vi "TCP Tester.vi"() -> ()   [LabVIEW 2019]
uses:
  <userlib>/Jet Engineering/JET_QSM/Code/Private/JET_QSM - Add State [String API].vi
  <userlib>/Jet Engineering/JET_QSM/Code/Private/JET_QSM_InvalidOption STYP.ctl
  Code/Shared/Map/Map.lvclass
panel:
  out "Recent states before Error (with tick counts) 3":string="0.167 sec ago: VI Initialize\n0.167 sec ago: Window Open\n0.110 sec ago: Control Update\n0.110 sec ago: Indicator Update\n0.000 sec ago: Error Handler\r\n"
  in  "Status 2":T1
  out "error out 2":errorcluster
  in  "Port":u16
  in  "IP Address":string
  out "Recent states before Error (with tick counts) 2":string="0.167 sec ago: VI Initialize\n0.167 sec ago: Window Open\n0.110 sec ago: Control Update\n0.110 sec ago: Indicator Update\n0.000 sec ago: Error Handler\r\n"
  in  "Status":T2
  out "error out":errorcluster
  in  "stop":bool
  in  "Send Button":bool
  out "Received Message":string
  in  "Message to Send":string
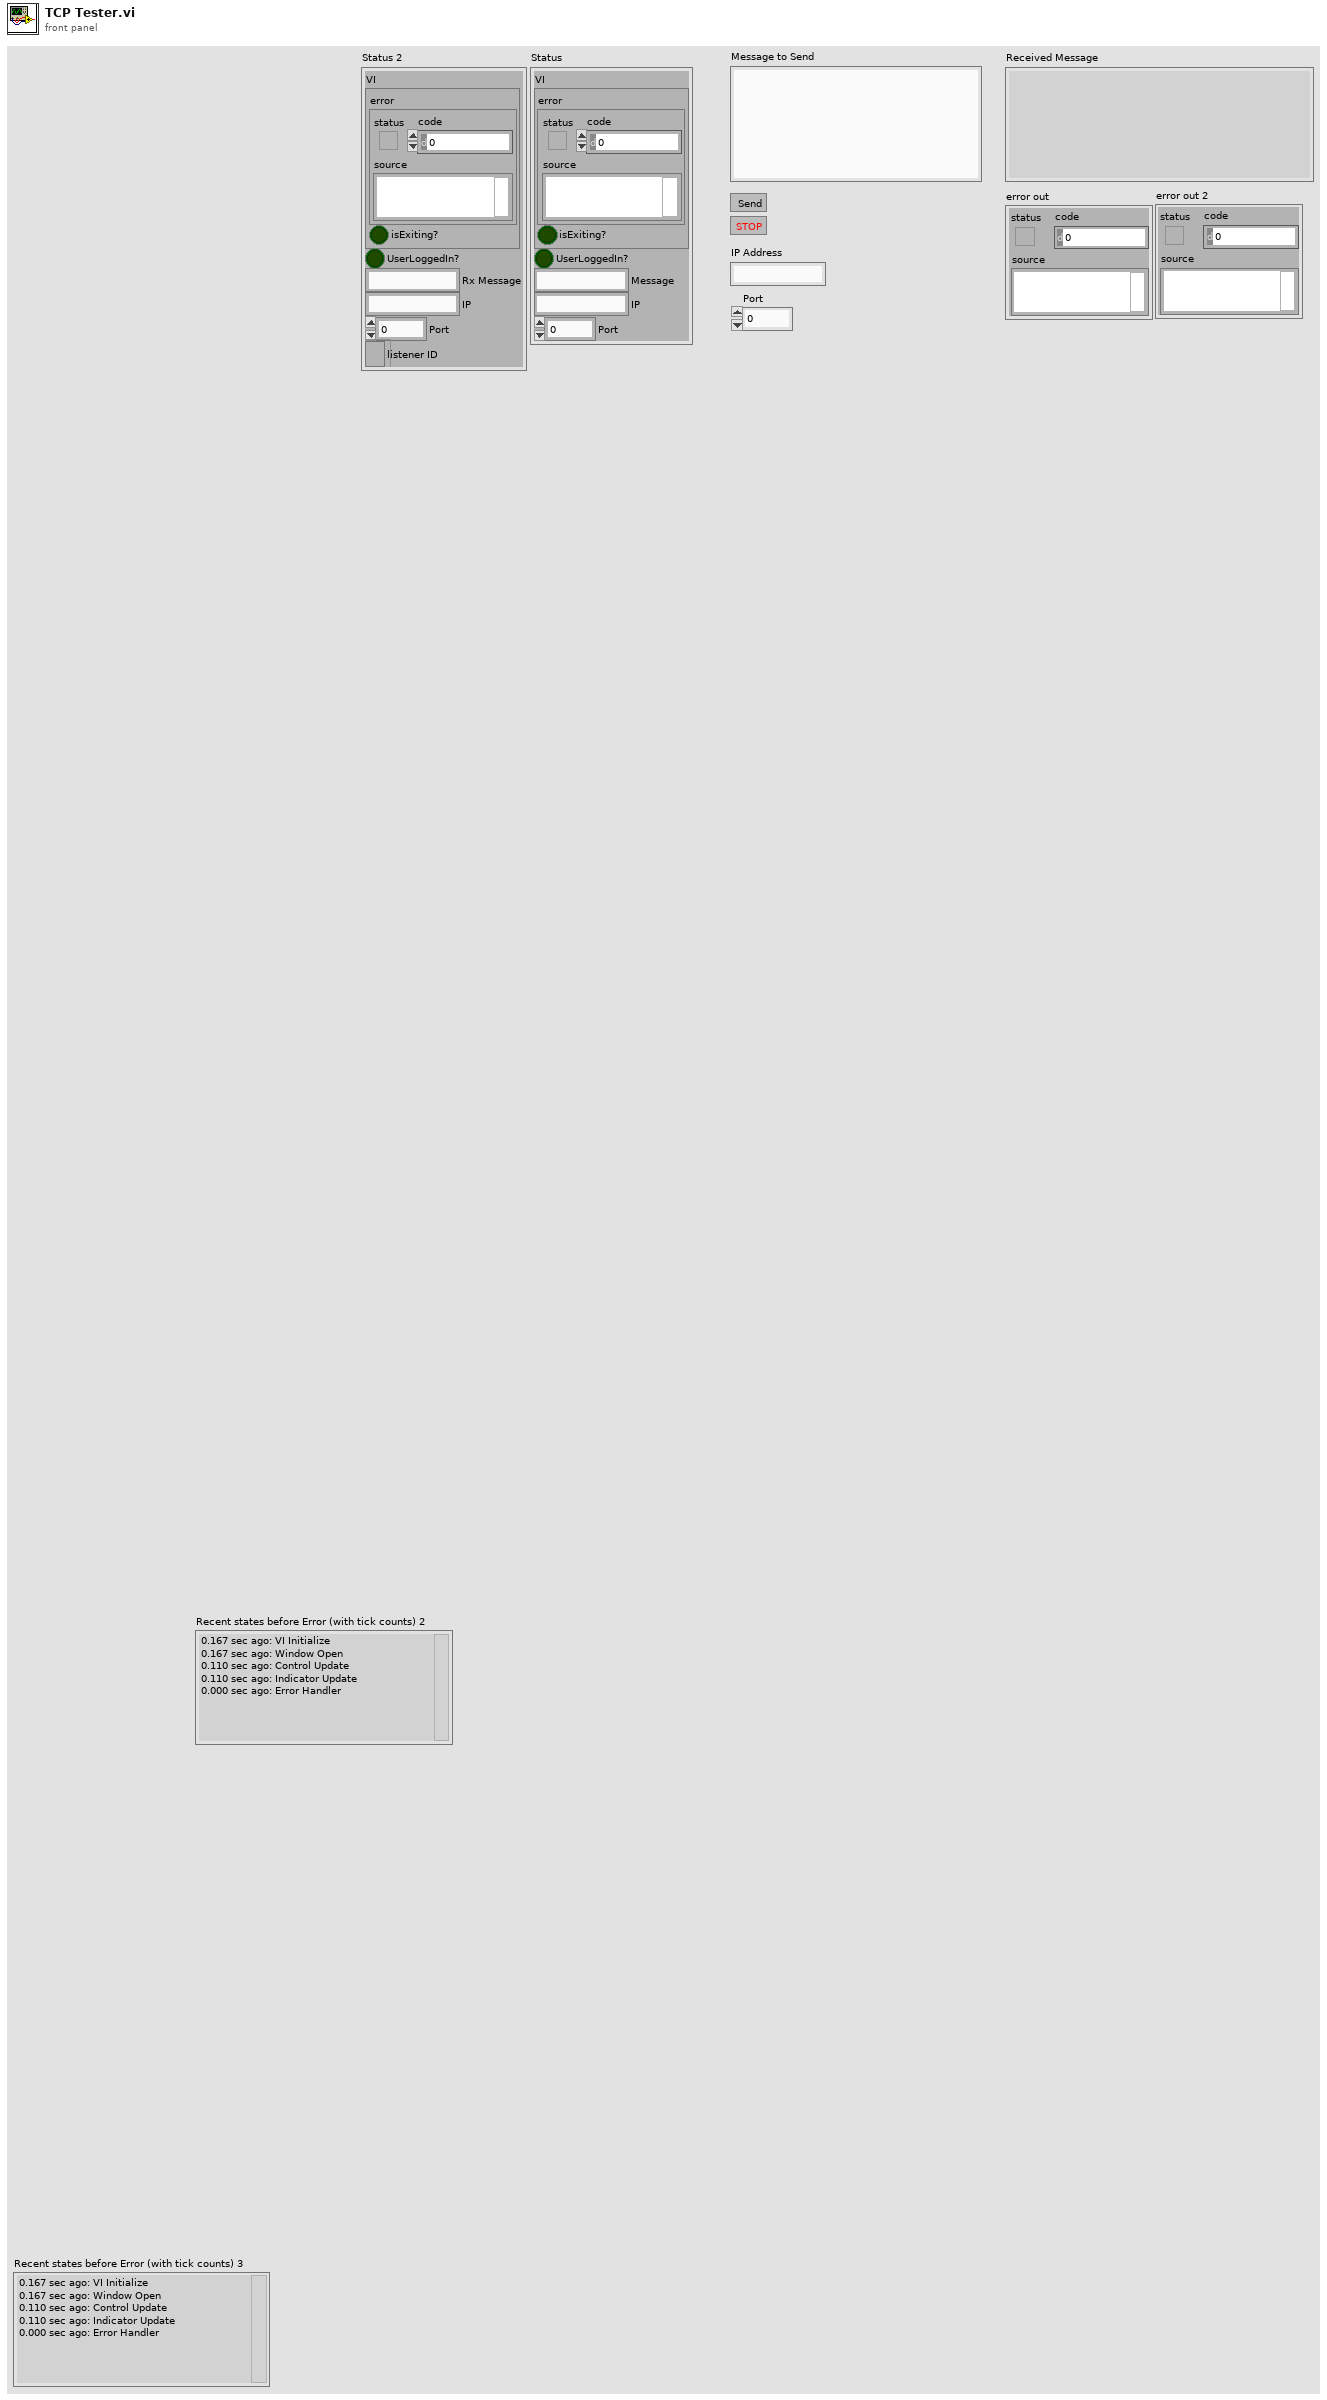
[diagram p1: front panel]
types:
  T1 = cluster{"VI":cluster{"error":errorcluster, "isExiting?":bool}, "UserLoggedIn?":bool, "Rx Message":string, "IP":string, "Port":u16, "listener ID":refnum<k5>}
  T2 = cluster{"VI":cluster{"error":errorcluster, "isExiting?":bool}, "UserLoggedIn?":bool, "Message":string, "IP":string, "Port":u16}
  T3 = typedef "JET_QSM_InvalidOption STYP.ctl" = enum16{"Ignore", "Dialog", "Error"}
  T4 = typedef "JET_QSM_Refnum STYP.ctl" = cluster{"state":cluster{"queue":refnum<queue>, "idle":string, "error":string, "STOP":string}, "debug":cluster{"enabled?":bool, "queue":refnum<queue>}, "Invalid.option":T3, "QSM.Name":string}
  T5 = enum32{"invalid app kind", "Development System", "Run Time System", "Student Edition", "Embedded LabVIEW", "Evaluation", "Custom"}
  T6 = typedef "JET_QSM_Element STYP.ctl" = cluster{"state":string, "data":variant, "comment":string}
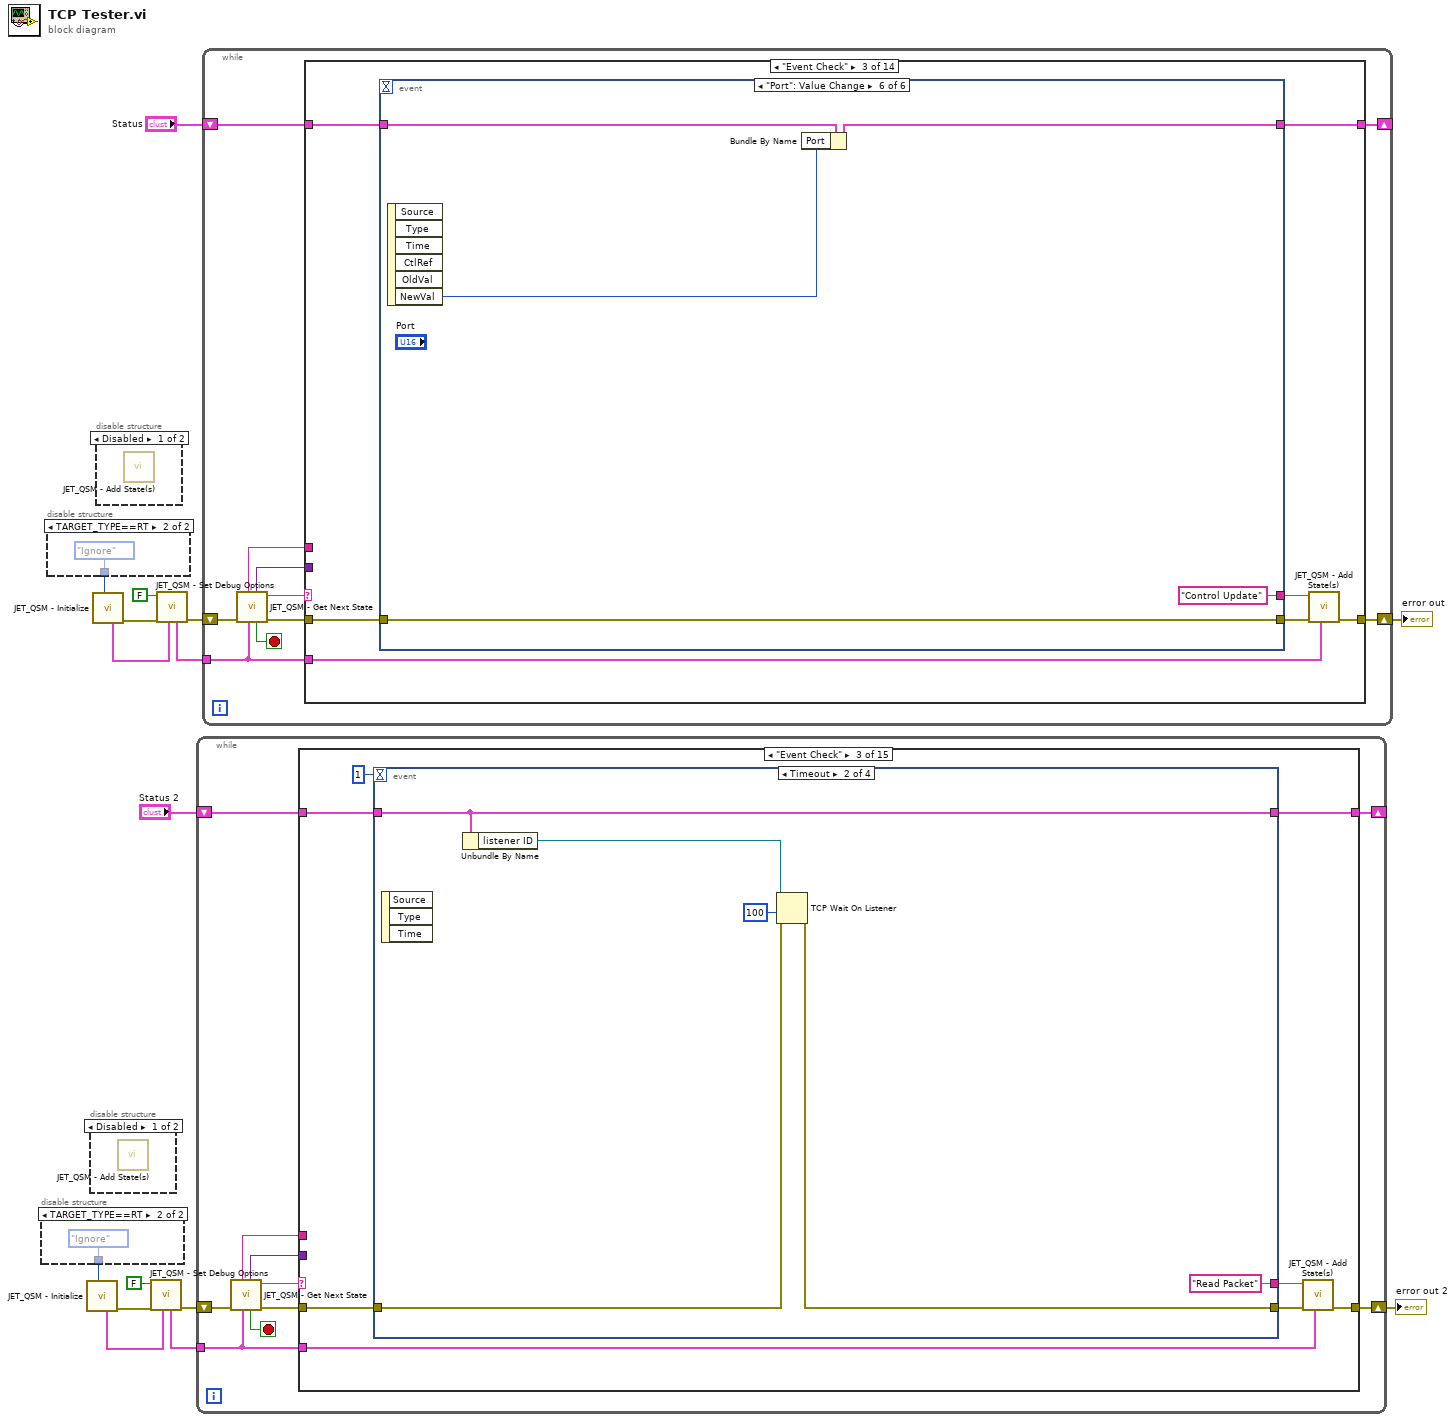
[diagram p0: block diagram]
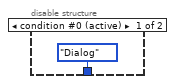
[diagram p2: hidden frame]
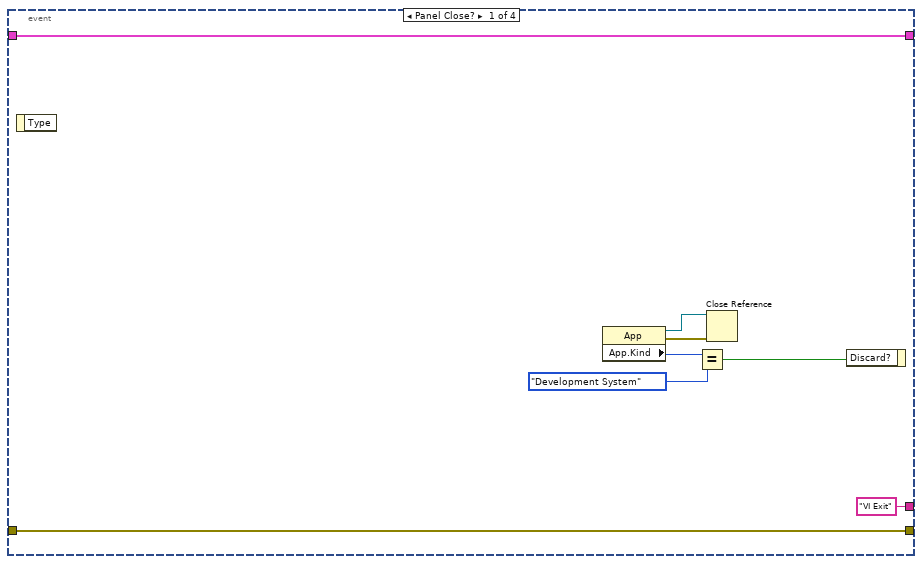
[diagram p6: hidden frame]
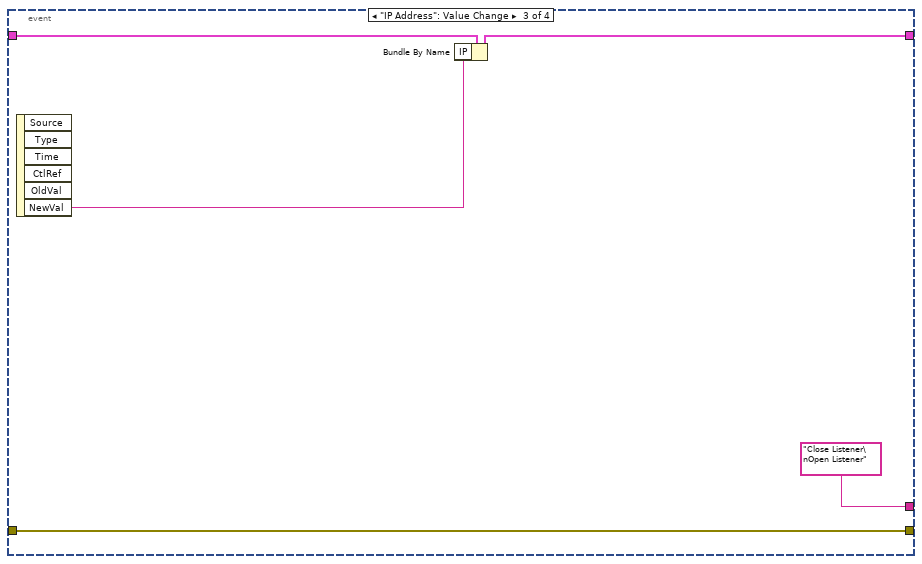
[diagram p7: hidden frame]
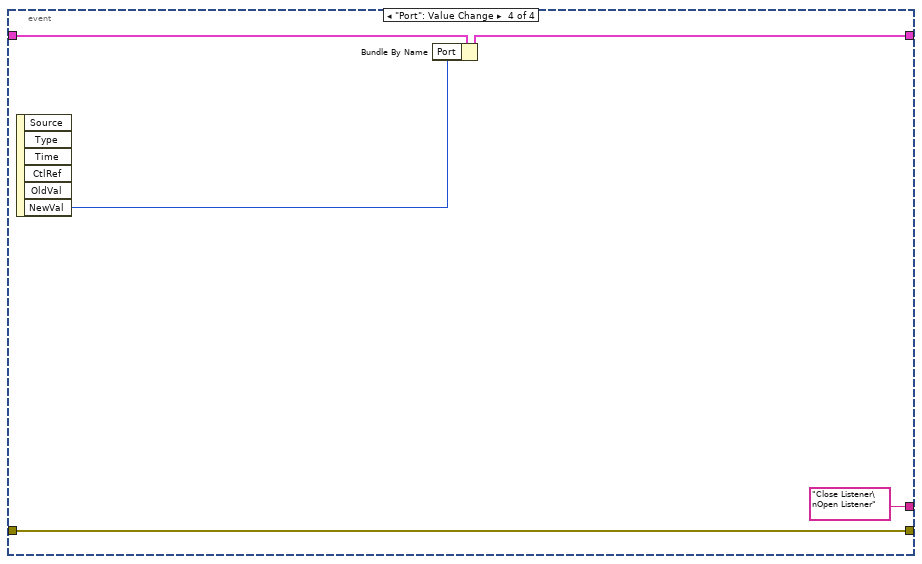
[diagram p8: hidden frame]
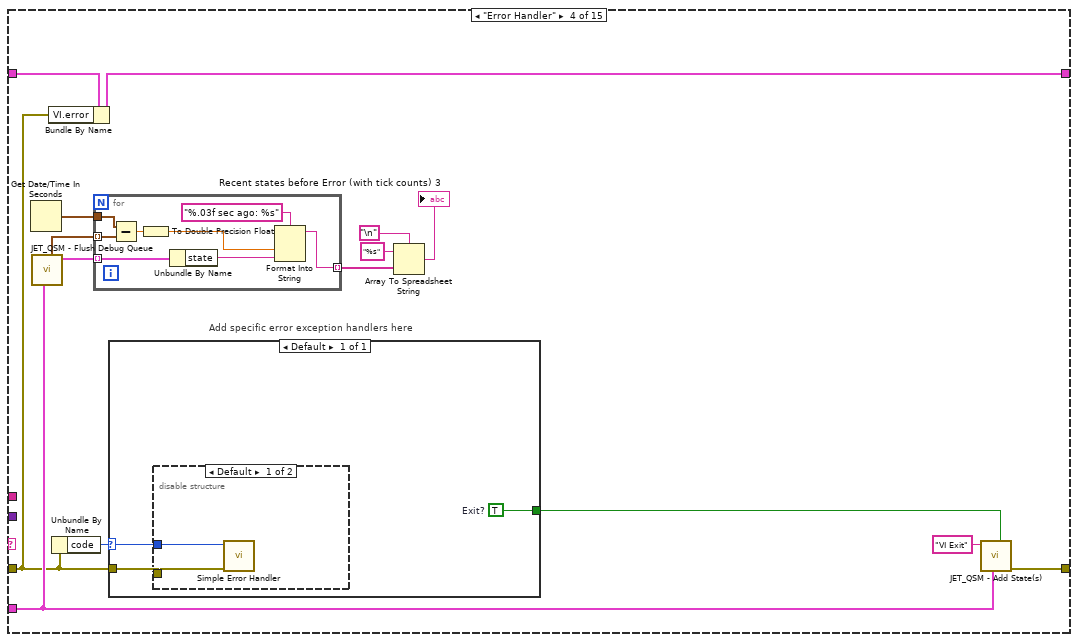
[diagram p9: hidden frame]
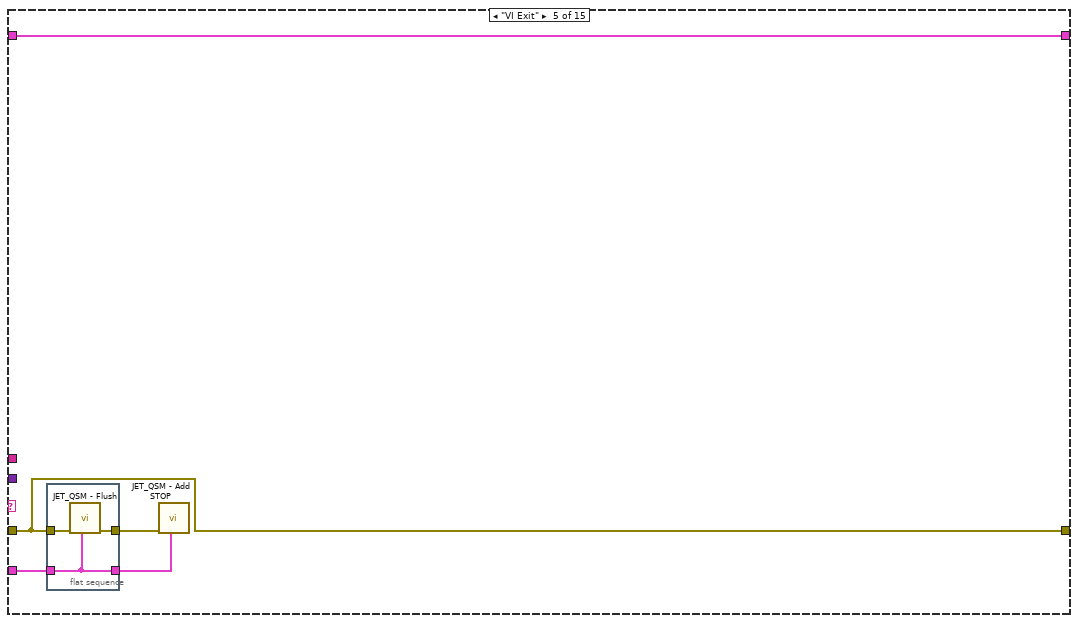
[diagram p11: hidden frame]
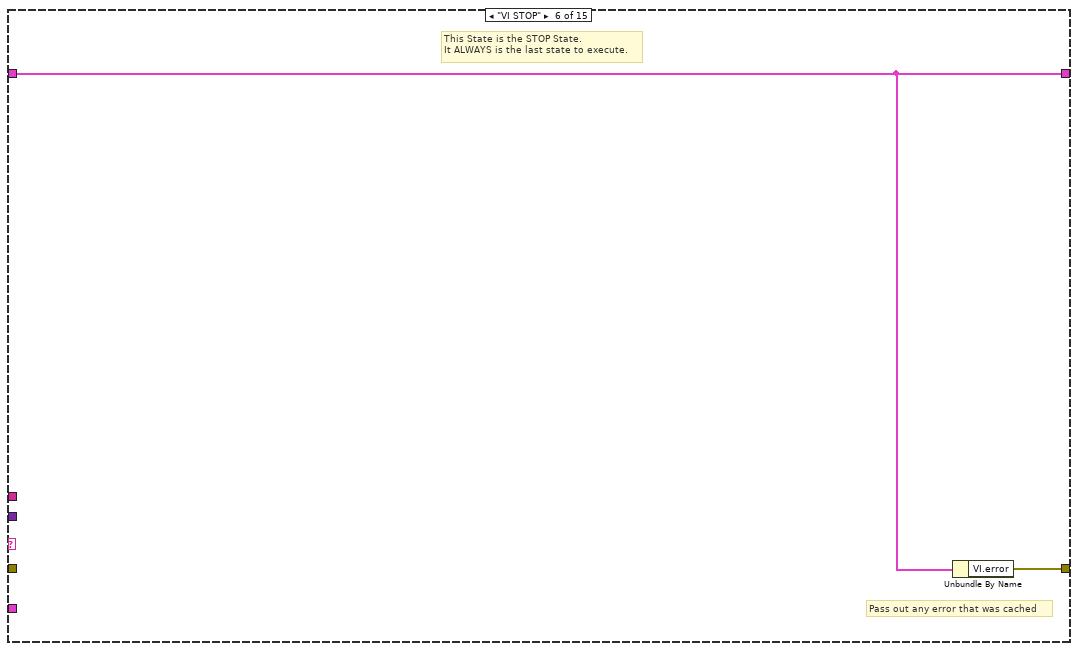
[diagram p12: hidden frame]
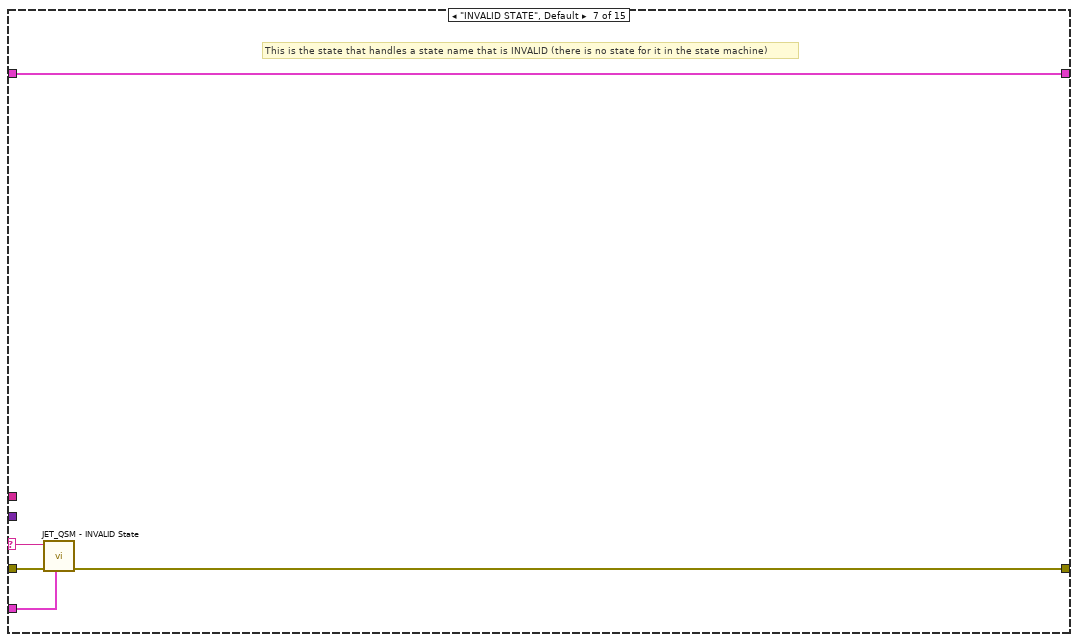
[diagram p13: hidden frame]
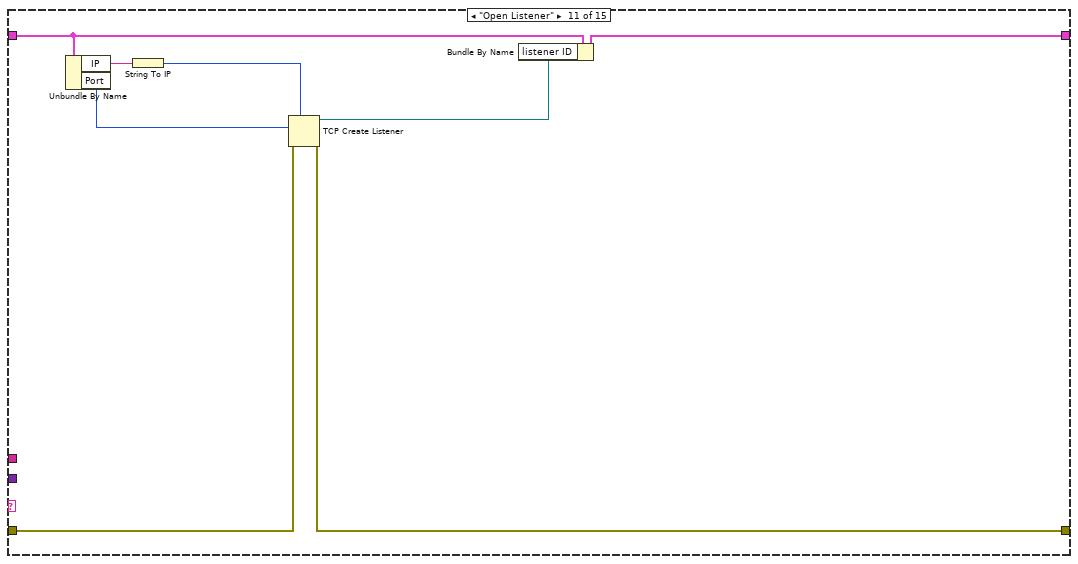
[diagram p17: hidden frame]
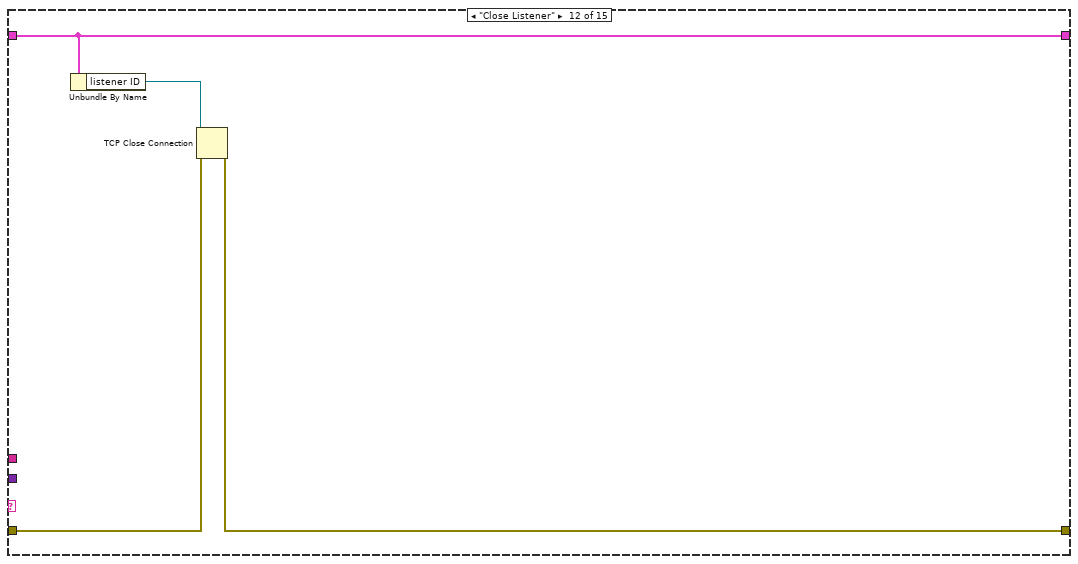
[diagram p18: hidden frame]
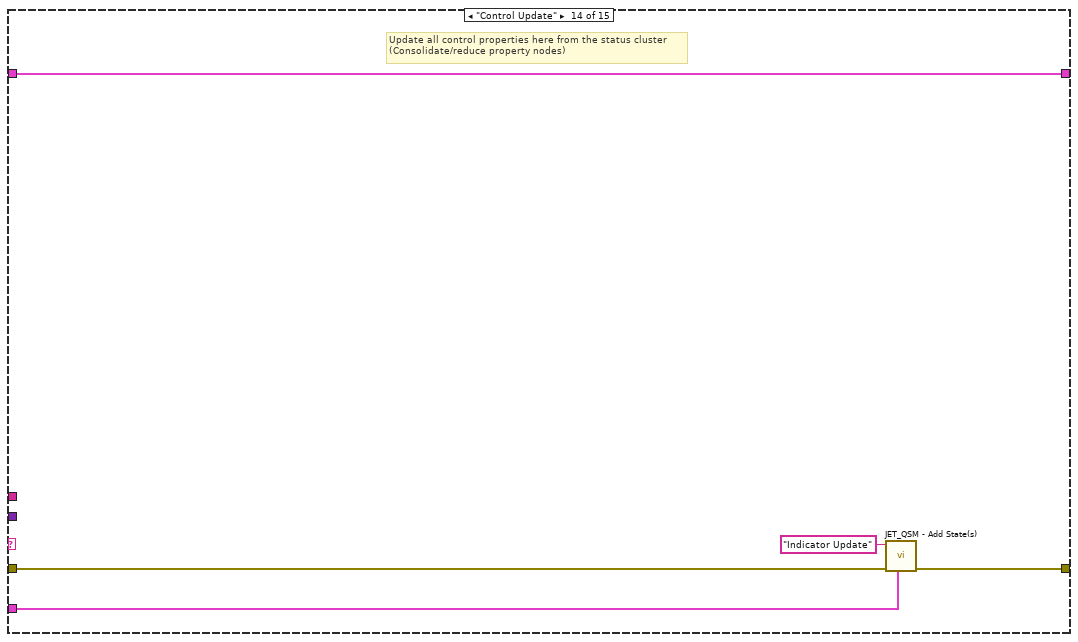
[diagram p20: hidden frame]
diagram:
  n1 = disable-structure shown="TARGET_TYPE==RT" {
    disable-tunnel: [JET_QSM_InvalidOption_STYP."Dialog" ("invalid state action (Dialog)") JET_QSM_InvalidOption_STYP."Ignore" ("invalid state action (Dialog)")] -> w8
    frame condition #0 (active) {
    }
    frame condition #1 {
    }
  }
  n2 = disable-structure shown="TARGET_TYPE==RT" {
    disable-tunnel: [JET_QSM_InvalidOption_STYP."Dialog" ("invalid state action (Dialog)") JET_QSM_InvalidOption_STYP."Ignore" ("invalid state action (Dialog)")] -> w16
    frame condition #0 (active) {
    }
    frame condition #1 {
    }
  }
  n3 = call <userlib>:"JET_QSM - Initialize.vi"("invalid state action (Dialog)"=w8) -> ("error out"=w1:errorcluster, "Jet_QSM refnum"=w4:T4)  [unwired: 9 in]
  n4 = disable-structure shown="Disabled" {
    frame Disabled {
      n5 = call-poly <userlib>:"JET_QSM - Add State(s).vi"() -> ()  [unwired: 11 in, 1 out]
    }
    frame Enabled {
    }
  }
  n6 = call <userlib>:"JET_QSM - Initialize.vi"("invalid state action (Dialog)"=w16) -> ("error out"=w9:errorcluster, "Jet_QSM refnum"=w12:T4)  [unwired: 9 in]
  n7 = disable-structure shown="Disabled" {
    frame Disabled {
      n8 = call-poly <userlib>:"JET_QSM - Add State(s).vi"() -> ()  [unwired: 11 in, 1 out]
    }
    frame Enabled {
    }
  }
  n9 = call <userlib>:"JET_QSM - Set Debug Options.vi"("Jet_QSM refnum"=w4, "error in (no error)"=w1, "debug.enabled? (F)"=FALSE) -> ("error out"=w2:errorcluster, "Jet_QSM ref"=w3:T4)  [unwired: 7 in]
  n10 = call <userlib>:"JET_QSM - Set Debug Options.vi"("Jet_QSM refnum"=w12, "error in (no error)"=w9, "debug.enabled? (F)"=FALSE) -> ("error out"=w10:errorcluster, "Jet_QSM ref"=w11:T4)  [unwired: 7 in]
  n11 = while {
    tunnel: w3 -> [w26]
    shift-right: [w24] -> _
    shift-left: "Status 2" -> [w25]
    shift-right: [w23] -> w7
    shift-left: w2 -> [w30]
    stop <- w27 stop-if-true
    n12 = call <userlib>:"JET_QSM - Get Next State.vi"("Jet_QSM refnum"=w26, "error in (no error)"=w30) -> ("error out"=w29:errorcluster, "state"=w28:string, "Stop Loop?"=w27:bool, "state data"=w22:variant, "state comment"=w21:string)  [unwired: 5 in]
    n13 = case shown="\"Event Check\"" w28 {
      selector: w28 -> [_ _ _ _ _ _ w107 _ _ _ _ _ _ _ _]
      tunnel: w29 -> [w31 w33 w42 w68 w99 _ w108 w110 w112 w114 w120 w124 w128 w131 w137]
      tunnel: w26 -> [_ _ w41 w73 w97 _ w106 _ _ _ _ _ _ w132 _]
      tunnel: w25 -> [w32 w34 w37 w69 w95 w103 w109 w111 w113 w115 w119 w127 w129 w134 w136]
      tunnel: [w32 w34 w36 w67 w95 w103 w109 w111 w113 w115 w123 w127 w129 w134 w136] -> w24
      tunnel: [w31 w33 w39 w74 w99 w104 w105 w110 w112 w114 w121 w125 w128 w130 w137] -> w23
      tunnel: w22 -> [_ _ _ _ _ _ _ _ _ _ _ _ _ _ _]
      tunnel: w21 -> [_ _ _ _ _ _ _ _ _ _ _ _ _ _ _]
      frame "------ Standard States ------" {
        # "Standard States are required states for a JET_QSM State Machine\n\nTheir names may be changed; use the Initialize function to specify the new names"
        # "This is a section header; the state is never expected to execute"
      }
      frame "VI Initialize" {
      }
      frame "Event Check" {
        n14 = event shown="[1] Timeout" {
          selector: _ -> [_ _ _ _]
          dyn-events: _ -> [_ _ _ _]
          timeout: 1 -> [_ _ _ _]
          tunnel: w42 -> [w44 w52 w60 w65]
          tunnel: ["VI Exit" ("state(s)") "Read Packet" ("state(s)") "Close Listener\nOpen Listener" ("state(s)") "Close Listener\nOpen Listener" ("state(s)")] -> w40
          tunnel: [w44 w53 w60 w65] -> w38
          tunnel: w37 -> [w43 w56 w61 w66]
          tunnel: [w43 w56 w58 w63] -> w36
          event Panel Close? {
            n15 = event-data() -> ()  [unwired: 1 in, 1 out]
            n16 = property class="App"() -> (reference out=w46:refnum<vi>, error out=w47:errorcluster, "App.Kind"=w50:T5)  [unwired: 2 in]
            n17 = Equal?(x=w50, y=T5."Development System") -> (x = y?=w48:bool)
            n18 = Close Reference(reference=w46, error in (no error)=w47) -> ()  [unwired: 1 out]
            n19 = event-data("Discard?"=w48) -> ()  [unwired: 1 in, 1 out]
          }
          event Timeout {
            n20 = event-data() -> ()  [unwired: 1 in, 3 out]
            n21 = Unbundle By Name(w56) -> ("listener ID"=w55:refnum<k5>)
            n22 = TCP Wait On Listener(8:w52, 9:100 ("timeout ms (wait forever: -1)"), 11:w55) -> (0:w53:errorcluster)  [unwired: 1 in, 4 out]
          }
          event "IP Address": Value Change {
            n23 = event-data() -> ("NewVal"=w57:string)  [unwired: 1 in, 5 out]
            n24 = Bundle By Name(cluster=w61, "IP"=w57) -> (w58:T1)
          }
          event "Port": Value Change {
            n25 = event-data() -> ("NewVal"=w62:u16)  [unwired: 1 in, 5 out]
            n26 = Bundle By Name(cluster=w66, "Port"=w62) -> (w63:T1)
          }
        }
        n27 = call-poly <userlib>:"JET_QSM - Add State(s).vi"("Jet_QSM refnum"=w41, "error in (no error)"=w38, "state(s)"=w40) -> ("error out"=w39:errorcluster)  [unwired: 8 in]
      }
      frame "Error Handler" {
        # "Add specific error exception handlers here"
        n28 = Get Date/Time In Seconds() -> (seconds since 1Jan1904=w77:timestamp)
        n29 = call <userlib>:"JET_QSM - Flush Debug Queue.vi"("Jet_QSM refnum"=w73) -> ("QSM Elements"=w75:T6[], "Timestamps"=w76:timestamp[])  [unwired: 8 in, 1 out]
        n30 = Bundle By Name(cluster=w69, "VI.error"=w68) -> (w67:T1)
        n31 = Unbundle By Name(w68) -> ("code"=w70:i32)
        n32 = for {
          tunnel: w75 -> [w89] mode=indexing
          tunnel: [w87] -> w79 mode=indexing
          tunnel: w77 -> [w84]
          tunnel: w76 -> [w85] mode=indexing
          n33 = Subtract(x=w84, y=w85) -> (x-y=w83:dbl)
          n34 = To Double Precision Float(number=w83) -> (double precision float=w82:dbl)
          n35 = Unbundle By Name(w89) -> ("state"=w88:string)
          n36 = Format Into String(format string="%.03f sec ago: %s", w82, w88) -> (resulting string=w87:string)  [unwired: 2 in, 1 out]
        }
        n37 = case shown="Default" w70 {
          selector: w70 -> [w91]
          tunnel: [w92] -> w71
          tunnel: w68 -> [w90]
          frame Default {
            w92 = TRUE  # Exit?
            n38 = disable-structure shown="Default" {
              disable-tunnel: w91 -> [w94 _]
              disable-tunnel: w90 -> [w93 _]
              frame condition #0 (active) {
                n39 = call <vilib>:"Simple Error Handler.vi"("error code (no error:0)"=w94, "error in (no error)"=w93) -> ()  [unwired: 3 in, 5 out]
              }
              frame condition #1 {
              }
            }
          }
        }
        n40 = Array To Spreadsheet String(delimiter (Tab)="\n", array=w79, 3:"%s" ("format string")) -> (spreadsheet string=→"Recent states before Error (with tick counts) 3":string)
        n41 = call-poly <userlib>:"JET_QSM - Add State(s).vi"("act? (T)"=w71, "Jet_QSM refnum"=w73, "state(s)"="VI Exit") -> ("error out"=w74:errorcluster)  [unwired: 8 in]
      }
      frame "VI Exit" {
        n42 = flat-sequence {
          tunnel: w99 -> [w102]
          tunnel: [w101] -> w98
          tunnel: w97 -> [w100]
          tunnel: [w100] -> w96
          frame #0 {
            n43 = call <userlib>:"JET_QSM - Flush.vi"("Jet_QSM ref"=w100, "error in (no error)"=w102) -> ("error out"=w101:errorcluster)  [unwired: 8 in, 1 out]
          }
        }
        n44 = call <userlib>:"JET_QSM - Add STOP.vi"("Jet_QSM refnum"=w96, "error in (no error)"=w98) -> ()  [unwired: 9 in, 1 out]
      }
      frame "VI STOP" {
        # "Pass out any error that was cached"
        # "This State is the STOP State.\nIt ALWAYS is the last state to execute."
        n45 = Unbundle By Name(w103) -> ("VI.error"=w104:errorcluster)
      }
      frame "INVALID STATE", Default {
        # "This is the state that handles a state name that is INVALID (there is no state for it in the state machine)"
        n46 = call <userlib>:"JET_QSM - INVALID State.vi"("Jet_QSM refnum"=w106, "error in (no error)"=w108, "state"=w107) -> ("error out"=w105:errorcluster)  [unwired: 8 in]
      }
      frame "------ Menu Commands ------" {
        # "This is a section header; the state is never expected to execute"
      }
      frame "------ Events  ------" {
        # "This is a section header; the state is never expected to execute"
      }
      frame "------ Actions  ------" {
        # "This is a section header; the state is never expected to execute"
      }
      frame "Open Listener" {
        n47 = Unbundle By Name(w119) -> ("IP"=w118:string, "Port"=w116:u16)
        n48 = String To IP(1:w118) -> (0:w117:u32)
        n49 = TCP Create Listener(7:w117, 8:w120, 10:w116) -> (0:w121:errorcluster, 3:w122:refnum<k5>)  [unwired: 2 in, 1 out]
        n50 = Bundle By Name(cluster=w119, "listener ID"=w122) -> (w123:T1)
      }
      frame "Close Listener" {
        n51 = Unbundle By Name(w127) -> ("listener ID"=w126:refnum<k5>)
        n52 = TCP Close Connection(connection ID=w126, error in (no error)=w124) -> (error out=w125:errorcluster)  [unwired: 1 in, 1 out]
      }
      frame "------ Window and Panel Control ------" {
        # "This is a section header; the state is never expected to execute"
      }
      frame "Control Update" {
        # "Update all control properties here from the status cluster\n(Consolidate/reduce property nodes)"
        n53 = call-poly <userlib>:"JET_QSM - Add State(s).vi"("Jet_QSM refnum"=w132, "error in (no error)"=w131, "state(s)"="Indicator Update") -> ("error out"=w130:errorcluster)  [unwired: 8 in]
      }
      frame "Indicator Update" {
        # "Update all indicator values here from the status cluster\n(Eliminate Local Variables)"
        n54 = Unbundle By Name(w136) -> ("Rx Message"=→"Received Message":string)
      }
    }
  }
  "error out 2" <- w7
  n55 = while {
    tunnel: w11 -> [w143]
    shift-right: [w141] -> _
    shift-left: "Status" -> [w142]
    shift-right: [w140] -> w15
    shift-left: w10 -> [w147]
    stop <- w144 stop-if-true
    n56 = call <userlib>:"JET_QSM - Get Next State.vi"("Jet_QSM refnum"=w143, "error in (no error)"=w147) -> ("error out"=w146:errorcluster, "state"=w145:string, "Stop Loop?"=w144:bool, "state data"=w139:variant, "state comment"=w138:string)  [unwired: 5 in]
    n57 = case shown="\"Event Check\"" w145 {
      selector: w145 -> [_ _ _ _ _ _ w228 _ _ _ _ _ _ _]
      tunnel: w146 -> [w148 w150 w158 w189 w220 _ w229 w231 w233 w235 w237 w255 w262 w266]
      tunnel: w143 -> [_ _ w157 w194 w218 _ w227 _ _ _ w240 _ w263 _]
      tunnel: w142 -> [w149 w151 w153 w190 w216 w224 w230 w232 w234 w236 w250 w256 w260 w265]
      tunnel: [w149 w151 w152 w188 w216 w224 w230 w232 w234 w236 w250 w256 w260 w265] -> w141
      tunnel: [w148 w150 w155 w195 w220 w225 w226 w231 w233 w235 w241 w255 w261 w266] -> w140
      tunnel: w139 -> [_ _ _ _ _ _ _ _ _ _ _ _ _ _]
      tunnel: w138 -> [_ _ _ _ _ _ _ _ _ _ _ _ _ _]
      frame "------ Standard States ------" {
        # "Standard States are required states for a JET_QSM State Machine\n\nTheir names may be changed; use the Initialize function to specify the new names"
        # "This is a section header; the state is never expected to execute"
      }
      frame "VI Initialize" {
      }
      frame "Event Check" {
        n58 = event shown="[5] \"Port\": Value Change" {
          selector: _ -> [_ _ _ _ _ _]
          dyn-events: _ -> [_ _ _ _ _ _]
          timeout: _ -> [_ _ _ _ _ _]
          tunnel: w158 -> [w160 w169 w172 w176 w181 w186]
          tunnel: ["VI Exit" ("state(s)") "Control Update" ("state(s)") "VI Exit" ("state(s)") "Send TCP" ("state(s)") "Control Update" ("state(s)") "Control Update" ("state(s)")] -> w156
          tunnel: [w160 w169 w172 w176 w181 w186] -> w154
          tunnel: w153 -> [w159 w171 w174 w177 w182 w187]
          tunnel: [w159 w168 w174 w177 w179 w184] -> w152
          event Panel Close? {
            n59 = event-data() -> ()  [unwired: 1 in, 1 out]
            n60 = property class="App"() -> (reference out=w162:refnum<vi>, error out=w163:errorcluster, "App.Kind"=w166:T5)  [unwired: 2 in]
            n61 = Equal?(x=w166, y=T5."Development System") -> (x = y?=w164:bool)
            n62 = Close Reference(reference=w162, error in (no error)=w163) -> ()  [unwired: 1 out]
            n63 = event-data("Discard?"=w164) -> ()  [unwired: 1 in, 1 out]
          }
          event "Message to Send": Value Change {
            n64 = event-data() -> ("NewVal"=w167:string)  [unwired: 1 in, 5 out]
            n65 = Bundle By Name(cluster=w171, "Message"=w167) -> (w168:T2)
          }
          event "stop": Value Change {
            n66 = event-data() -> ()  [unwired: 1 in, 6 out]
          }
          event "Send Button": Value Change {
            n67 = event-data() -> ()  [unwired: 1 in, 6 out]
          }
          event "IP Address": Value Change {
            n68 = event-data() -> ("NewVal"=w178:string)  [unwired: 1 in, 5 out]
            n69 = Bundle By Name(cluster=w182, "IP"=w178) -> (w179:T2)
          }
          event "Port": Value Change {
            n70 = event-data() -> ("NewVal"=w183:u16)  [unwired: 1 in, 5 out]
            n71 = Bundle By Name(cluster=w187, "Port"=w183) -> (w184:T2)
          }
        }
        n72 = call-poly <userlib>:"JET_QSM - Add State(s).vi"("Jet_QSM refnum"=w157, "error in (no error)"=w154, "state(s)"=w156) -> ("error out"=w155:errorcluster)  [unwired: 8 in]
      }
      frame "Error Handler" {
        # "Add specific error exception handlers here"
        n73 = Get Date/Time In Seconds() -> (seconds since 1Jan1904=w198:timestamp)
        n74 = call <userlib>:"JET_QSM - Flush Debug Queue.vi"("Jet_QSM refnum"=w194) -> ("QSM Elements"=w196:T6[], "Timestamps"=w197:timestamp[])  [unwired: 8 in, 1 out]
        n75 = Bundle By Name(cluster=w190, "VI.error"=w189) -> (w188:T2)
        n76 = Unbundle By Name(w189) -> ("code"=w191:i32)
        n77 = for {
          tunnel: w196 -> [w210] mode=indexing
          tunnel: [w208] -> w200 mode=indexing
          tunnel: w198 -> [w205]
          tunnel: w197 -> [w206] mode=indexing
          n78 = Subtract(x=w205, y=w206) -> (x-y=w204:dbl)
          n79 = To Double Precision Float(number=w204) -> (double precision float=w203:dbl)
          n80 = Unbundle By Name(w210) -> ("state"=w209:string)
          n81 = Format Into String(format string="%.03f sec ago: %s", w203, w209) -> (resulting string=w208:string)  [unwired: 2 in, 1 out]
        }
        n82 = case shown="Default" w191 {
          selector: w191 -> [w212]
          tunnel: [w213] -> w192
          tunnel: w189 -> [w211]
          frame Default {
            w213 = TRUE  # Exit?
            n83 = disable-structure shown="Default" {
              disable-tunnel: w212 -> [w215 _]
              disable-tunnel: w211 -> [w214 _]
              frame condition #0 (active) {
                n84 = call <vilib>:"Simple Error Handler.vi"("error code (no error:0)"=w215, "error in (no error)"=w214) -> ()  [unwired: 3 in, 5 out]
              }
              frame condition #1 {
              }
            }
          }
        }
        n85 = Array To Spreadsheet String(delimiter (Tab)="\n", array=w200, 3:"%s" ("format string")) -> (spreadsheet string=→"Recent states before Error (with tick counts) 2":string)
        n86 = call-poly <userlib>:"JET_QSM - Add State(s).vi"("act? (T)"=w192, "Jet_QSM refnum"=w194, "state(s)"="VI Exit") -> ("error out"=w195:errorcluster)  [unwired: 8 in]
      }
      frame "VI Exit" {
        n87 = flat-sequence {
          tunnel: w220 -> [w223]
          tunnel: [w222] -> w219
          tunnel: w218 -> [w221]
          tunnel: [w221] -> w217
          frame #0 {
            n88 = call <userlib>:"JET_QSM - Flush.vi"("Jet_QSM ref"=w221, "error in (no error)"=w223) -> ("error out"=w222:errorcluster)  [unwired: 8 in, 1 out]
          }
        }
        n89 = call <userlib>:"JET_QSM - Add STOP.vi"("Jet_QSM refnum"=w217, "error in (no error)"=w219) -> ()  [unwired: 9 in, 1 out]
      }
      frame "VI STOP" {
        # "Pass out any error that was cached"
        # "This State is the STOP State.\nIt ALWAYS is the last state to execute."
        n90 = Unbundle By Name(w224) -> ("VI.error"=w225:errorcluster)
      }
      frame "INVALID STATE", Default {
        # "This is the state that handles a state name that is INVALID (there is no state for it in the state machine)"
        n91 = call <userlib>:"JET_QSM - INVALID State.vi"("Jet_QSM refnum"=w227, "error in (no error)"=w229, "state"=w228) -> ("error out"=w226:errorcluster)  [unwired: 8 in]
      }
      frame "------ Menu Commands ------" {
        # "This is a section header; the state is never expected to execute"
      }
      frame "------ Events  ------" {
        # "This is a section header; the state is never expected to execute"
      }
      frame "------ Actions  ------" {
        # "This is a section header; the state is never expected to execute"
      }
      frame "Send TCP" {
        n92 = Unbundle By Name(w250) -> ("IP"=w249:string, "Port"=w248:u16, "Message"=w246:string)
        n93 = call-dynamic "Write Board String.vi"("Board String"=w246, "Map in"=refnum<class "Map.lvclass"> refnum) -> ("error out"=w244:errorcluster, "Map out"=w245:refnum<class "Map.lvclass">)  [unwired: 8 in]
        n94 = call-dynamic "Packet Encode.vi"("error in (no error)"=w244, "Map in"=w245) -> ("Data"=w243:u8[])  [unwired: 7 in, 2 out]
        n95 = Byte Array To String(unsigned byte array=w243) -> (string=w242:string)
        n96 = TCP Open Connection(address=w249, remote port or service name=w248, error in (no error)=w237) -> (connection ID=w254:refnum<k5>, error out=w251:errorcluster)  [unwired: 2 in]
        n97 = TCP Write(connection ID=w254, data in=w242, error in (no error)=w251) -> (connection ID out=w253:refnum<k5>, error out=w252:errorcluster)  [unwired: 1 in, 1 out]
        n98 = TCP Close Connection(connection ID=w253, error in (no error)=w252) -> (error out=w238:errorcluster)  [unwired: 1 in, 1 out]
        n99 = call-poly <userlib>:"JET_QSM - Add State(s).vi"("Jet_QSM refnum"=w240, "error in (no error)"=w238, "state(s)"="Wait for Packet") -> ("error out"=w241:errorcluster)  [unwired: 8 in]
      }
      frame "------ Window and Panel Control ------" {
        # "This is a section header; the state is never expected to execute"
      }
      frame "Control Update" {
        # "Update all control properties here from the status cluster\n(Consolidate/reduce property nodes)"
        n100 = Unbundle By Name(w260) -> ("Message"=w259:string, "IP"=w258:string, "Port"=w257:u16)
        n101 = local write "IP Address"(w258) -> ()
        n102 = local write "Port"(w257) -> ()
        n103 = local write "Message to Send"(w259) -> ()
        n104 = call-poly <userlib>:"JET_QSM - Add State(s).vi"("Jet_QSM refnum"=w263, "error in (no error)"=w262, "state(s)"="Indicator Update") -> ("error out"=w261:errorcluster)  [unwired: 8 in]
      }
      frame "Indicator Update" {
        # "Update all indicator values here from the status cluster\n(Eliminate Local Variables)"
      }
    }
  }
  "error out" <- w15
